vi "Construct - Input.vi"(4 "extension":string, 6 "file name format":string="Log %<%Y-%m-%d %H%M%S>T", 7 "Max File Size (MB)":dbl=512.0, 9 "Name":string, 10 "Level":T1=enum."DEBUG", 11 "log location":path) -> (0 "error out":errorcluster, 3 "SQLite Database out":refnum<class "SQLite Database.lvclass">)   [LabVIEW 2019, in "TSC Event Logger.lvlib" / "SQLite Database.lvclass"]
uses:
  SQLite Database.lvclass
  C:/Development/Reuse-libraries/Event Logger/Log Sinks/Log Sinks.lvclass
  Log/Event Level.ctl
  Layouts/DBLayout/DBLayout.lvclass
  C:/Development/Reuse-libraries/Event Logger/Layouts/Layout.lvclass
  SQLite Database.lvclass/SQLite Database.ctl
  Log Sinks.lvclass/Log Sinks.ctl
  Log Sinks.lvclass
  TSC Event Logger.lvlib
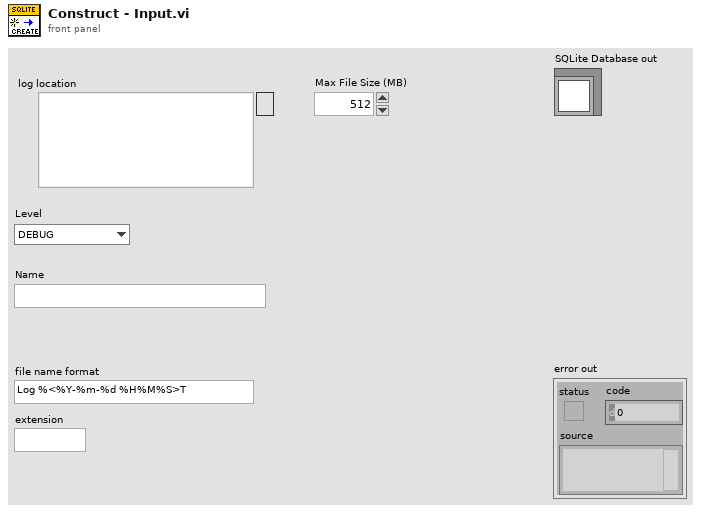
[diagram p1: front panel]
types:
  T1 = typedef "TSC Event Logger.lvlib/Event Level.ctl" = enum16{"OFF", "TRACE", "DEBUG", "INFO", "WARN", "ERROR", "FATAL"}
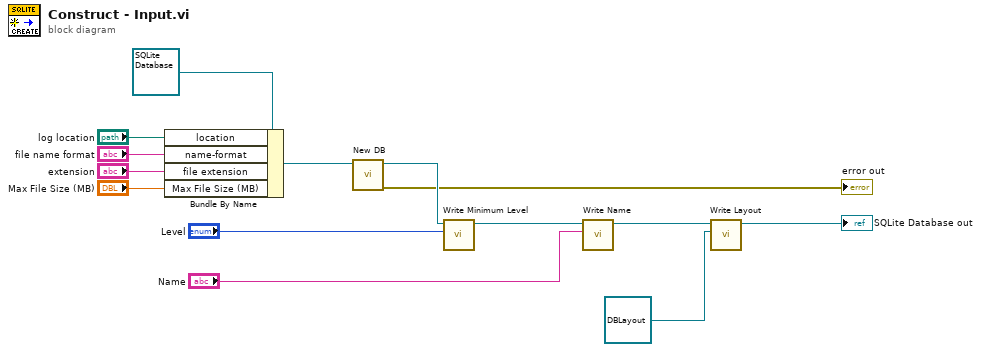
[diagram p0: block diagram]
diagram:
  n1 = Bundle By Name(cluster=refnum<class "SQLite Database.lvclass"> refnum ("TSC Event Logger.lvlib:SQLite Database.lvclass"), "location"="log location", "name-format"="file name format", "file extension"="extension", "Max File Size (MB)"="Max File Size (MB)") -> (w9:refnum<class "SQLite Database.lvclass">)
  n2 = call "New DB.vi"("SQLite Database in"=w9) -> ("error out"=→"error out":errorcluster, "SQLite Database out"=w8:refnum<class "SQLite Database.lvclass">)  [unwired: 9 in]
  n3 = call "Write Minimum Level.vi"("Level"="Level", "Log Sinks in"=w8) -> ("Log Sinks out"=w5:refnum<class "SQLite Database.lvclass">)  [unwired: 9 in]
  n4 = call "Write Name.vi"("Name"="Name", "Log Sinks in"=w5) -> ("Log Sinks out"=w6:refnum<class "SQLite Database.lvclass">)  [unwired: 9 in]
  n5 = call "Write Layout.vi"("Layout"=refnum<class "DBLayout.lvclass"> refnum ("TSC Event Logger.lvlib:DBLayout.lvclass"), "Log Sinks in"=w6) -> ("Log Sinks out"=→"SQLite Database out":refnum<class "SQLite Database.lvclass">)  [unwired: 9 in]
